vi "OrthogonalMatchingPursuit.vi"(8 "error in":errorcluster) -> (0 "error out":errorcluster, 3 "out":refnum<class "OrthogonalMatchingPursuit.lvclass">)   [LabVIEW 2020]
doc: "Orthogonal Matching Pursuit model (OMP).\n\n Read more in the :ref:`User Guide <omp>`.\n\n Parameters\n ----------\n n_nonzero_coefs : int, default=None\n Desired number of non-zero entries in the solution. If None (by\n default) this value is set to 10% of n_features.\n\n tol : float, default=None\n Maximum norm of the residual. If not None, overrides n_nonzero_coefs.\n\n fit_intercept : bool, default=True\n whether to calculate the intercept for this model. If set\n to false, no intercept will be used in calculations\n (i.e. data is expected to be centered).\n\n normalize : bool, default=True\n This parameter is ignored when ``fit_intercept`` is set to False.\n If True, the regressors X will be normalized before regression by\n subtracting the mean and dividing by the l2-norm.\n If you wish to standardize, please use\n :class:`~sklearn.preprocessing.StandardScaler` before calling ``fit``\n on an estimator with ``normalize=False``.\n\n precompute : 'auto' or bool, default='auto'\n Whether to use a precomputed Gram and Xy matrix to speed up\n calculations. Improves performance when :term:`n_targets` or\n :term:`n_samples` is very large. Note that if you already have such\n matrices, you can pass them directly to the fit method.\n\n Attributes\n ----------\n coef_ : ndarray of shape (n_features,) or (n_targets, n_features)\n Parameter vector (w in the formula).\n\n intercept_ : float or ndarray of shape (n_targets,)\n Independent term in decision function.\n\n n_iter_ : int or array-like\n Number of active features across every target.\n\n n_nonzero_coefs_ : int\n The number of non-zero coefficients in the solution. If\n `n_nonzero_coefs` is None and `tol` is None this value is either set\n to 10% of `n_features` or 1, whichever is greater.\n\n \nAvailable methods:\nGet Attributes\nGet Params\nSet Params"
uses:
  OrthogonalMatchingPursuit.lvclass
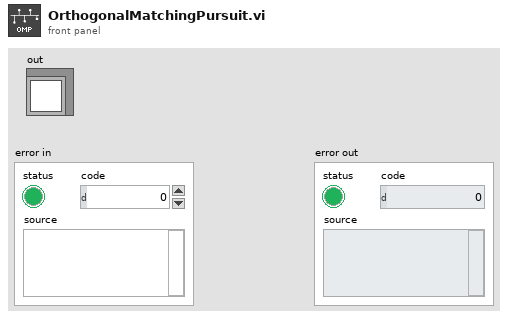
[diagram p1: front panel]
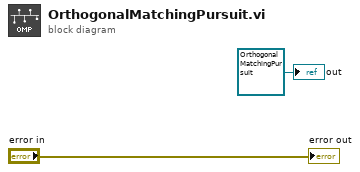
[diagram p0: block diagram]
diagram:
  "out" <- refnum<class "OrthogonalMatchingPursuit.lvclass"> refnum ("model")
  "error out" <- "error in"
